vi "PMT_plus_Kiethley2450_and_2410.vi"() -> ()   [LabVIEW 2024]
uses:
  <vilib>/Analysis/NI_AALBase.lvlib
  <vilib>/Analysis/1siggen.llb/Ramp Pattern by Delta.vi
  Keithley 2450/Keithley 2450.lvlib
  archive/Keithley 24XX/Keithley 24XX.lvlib
  <vilib>/Utility/file.llb/Write Delimited Spreadsheet (DBL).vi
  <vilib>/Utility/file.llb/Write Delimited Spreadsheet (string).vi
panel:
  out "Set voltage 2410":dbl
  out "current 2450":dbl format="%e"
  out "actual voltage 2410":dbl format="%0.2f"
  out "current 2410":dbl format="%e"
  in  "Compliance  Level 24210 (0.1)":dbl=0.1
  in  "VISA resource name 2410":refnum<visa-resource-name>
  out "Serial Configuration":T1={"Baud Rate"=9600, "Parity"=0, "Data Bits"=8, "Stop Bits"=10, "Flow Control"=0} {"Flow Control" items=["None", "XON/XOFF", "RTS/CTS", "XON/XOFF & RTS/CTS", "DTR/DSR", "XON/XOFF & DTR/DSR"]; "Stop Bits" items=["1.0"=10, "1.5"=15, "2.0"=20]; "Data Bits" items=["7"=7, "8"=8]; "Parity" items=["None", "Odd", "Even", "Mark", "Space"]; "Baud Rate" items=["300"=300, "600"=600, "1200"=1200, "2400"=2400, "4800"=4800, "9600"=9600, "19200"=19200]}
  in  "Use PMT?":bool=TRUE
  out "XY Graph":cluster{dbl[], dbl[]}(graph)
  out "Actual Voltage 2450":dbl
  in  "Num Current Meas":i32=6
  in  "Path":path
  out "error out":errorcluster
  in  "error in (no error)":errorcluster
  in  "VISA resource name":refnum<visa-resource-name>
  out "Set Voltage 2450":dbl
  in  "Step Size (V)":dbl=0.1 format="%#_13g"
  in  "Max V":dbl format="%#_13g"
  in  "Start V":dbl format="%#_13g"
  in  "Source Limit Level (0.1)":dbl=5e-08
  out "standard deviation":dbl
  out "mean":dbl
  out "data":u32[](array[numeric])
  out "OLD":bool
  out "DB":u32[](array[numeric])
  out "Overload":i32
  out "Gate Number":i32
  in  "Correction":bool=TRUE
  out "Num Gates Read":i32
  out "Gate Time Read":i32 caption="Gate time Read"
  out "Num Gates Set":i32=20
  out "Gate Time Set":i32=200
  out "PowerD":i32 caption="Power\nRead Data"
  out "Handle Number":i32
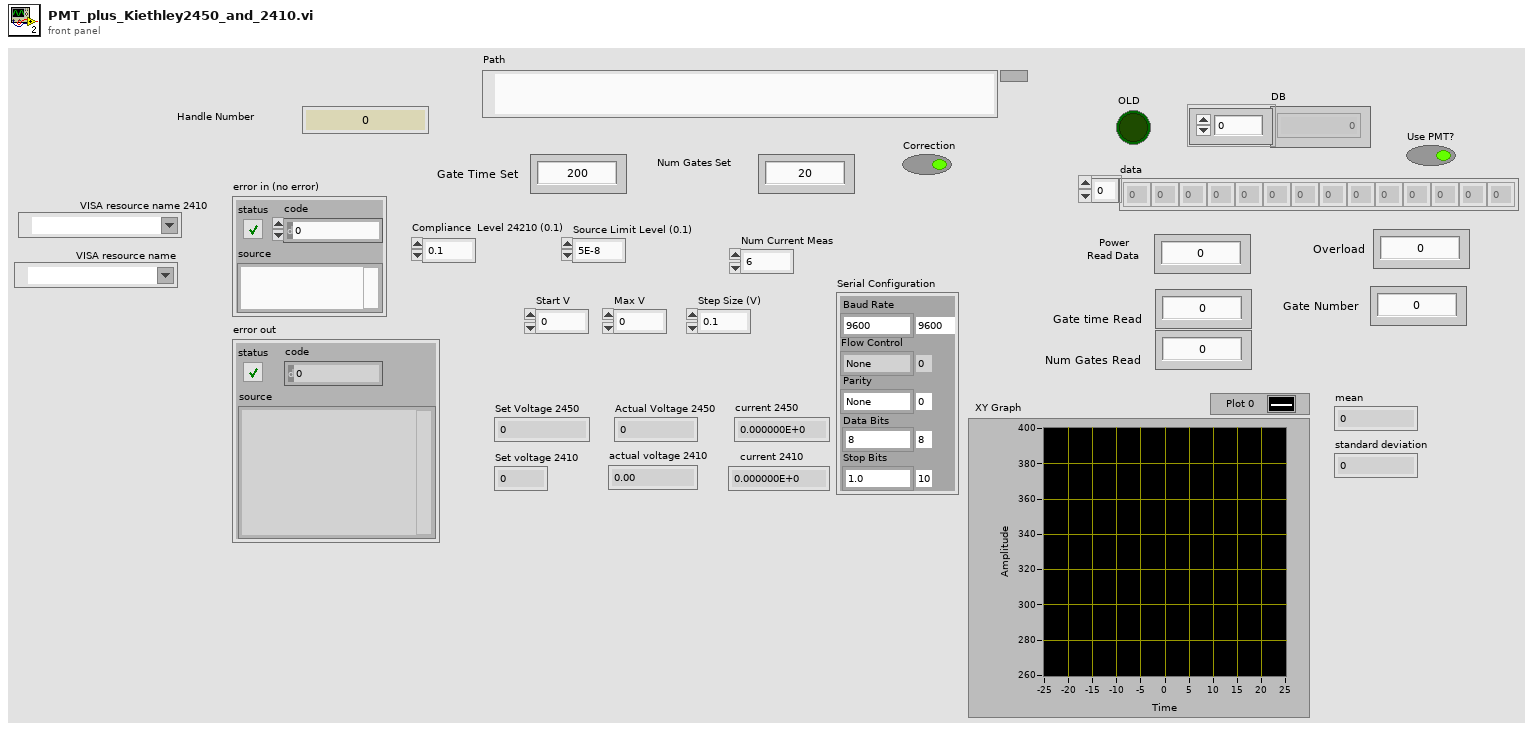
[diagram p1: front panel]
types:
  T1 = cluster{"Baud Rate":u32, "Parity":u16, "Data Bits":u16, "Stop Bits":u16, "Flow Control":u16}
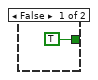
[diagram p2: hidden frame]
diagram:
  n1 = flat-sequence {
    tunnel: [w25] -> w5
    tunnel: [w14] -> w4
    tunnel: [w13] -> w3
    tunnel: ["Path"] -> w1
    tunnel: w5 -> [w43]
    tunnel: w4 -> [w42]
    tunnel: w3 -> [w41]
    tunnel: [w40] -> w2
    tunnel: w1 -> [w39]
    tunnel: w2 -> [w478]
    frame #0 {
      w8 = -1.0
      # "open PMT and turn on power"
      n2 = call "Open.vi"("Serial Number"="30430219") -> ("Handle Number"=w29:i32)  [unwired: 9 in, 1 out]
      "Handle Number" <- w29
      n3 = Boolean To (0,1)(Boolean="Use PMT?") -> (0, 1=w30:i16)
      n4 = call "Read HV.vi"("handle"=w29) -> ("HV out"=w28:i32, "handle out"=w32:i32)  [unwired: 8 in, 1 out]
      n5 = local write "PowerD"(w28) -> ()
      n6 = Multiply(x="Step Size (V)", y=w8) -> (x*y=w6:dbl)
      n7 = Multiply(x="Max V", y=w8) -> (x*y=w16:dbl)
      n8 = To Long Integer(number=w30) -> (32bit integer=w31:i32)
      n9 = call "Set HV.vi"("HV"=w31, "handle"=w32) -> ("handle out"=w34:i32)  [unwired: 8 in, 1 out]
      n10 = call-poly <vilib>:"Ramp Pattern.vi"("start"="Start V", "end"="Max V", "delta"="Step Size (V)") -> ("samples"=w21:i32, "Ramp Pattern"=w18:dbl[])  [unwired: 6 in, 1 out]
      n11 = call-poly <vilib>:"Ramp Pattern.vi"("start"="Max V", "end"=w16, "delta"=w6) -> ("samples"=w22:i32, "Ramp Pattern"=w19:dbl[])  [unwired: 6 in, 1 out]
      n12 = call-poly <vilib>:"Ramp Pattern.vi"("start"=w16, "end"="Start V", "delta"="Step Size (V)") -> ("samples"=w24:i32, "Ramp Pattern"=w20:dbl[])  [unwired: 6 in, 1 out]
      n13 = Add(x=w21, y=w22) -> (x+y=w23:i32)
      n14 = Build Array (concatenate)(w18, w19, w20) -> (w14:dbl[])
      n15 = Build Array("# SetVoltage2450(V) ActualVoltage2450(V) CountsMean CountsStd Current2450(uA) Current2450Std(uA) Current2410(uA) Current2410Std(uA)") -> (w10:string[])
      n16 = call "Read HV.vi"("handle"=w34) -> ("HV out"=w33:i32, "handle out"=w25:i32)  [unwired: 8 in, 1 out]
      n17 = local write "PowerD"(w33) -> ()
      n18 = Add(x=w23, y=w24) -> (x+y=w13:i32)
      n19 = call-poly <vilib>:"Write Delimited Spreadsheet.vi"("file path (dialog if empty)"="Path", "1D data"=w10, "append to file? (new file:F)"=TRUE) -> ()  [unwired: 11 in, 2 out]
    }
    frame #1 {
      w37 = 0
      w38 = 0
      n20 = Initialize Array(w37, w37) -> (w36:i32[])
      n21 = Initialize Array(w38, w38) -> (w35:i32[])
      n22 = for {
        N: w41 -> [_]
        tunnel: w42 -> [w79] mode=indexing
        tunnel: w43 -> [w78]
        tunnel: [w77] -> w40
        tunnel: w39 -> [w76]
        shift-right: [w63] -> _
        shift-left: w35 -> [w71]
        shift-right: [w64] -> _
        shift-left: w36 -> [w70]
        n23 = flat-sequence {
          tunnel: w70 -> [w126]
          tunnel: w71 -> [w127]
          tunnel: w79 -> [w80]
          tunnel: [w80] -> w62
          tunnel: [w127] -> w60
          tunnel: [w126] -> w58
          tunnel: [w110] -> w56
          tunnel: [w109] -> w54
          tunnel: [w93] -> w50
          tunnel: [w92] -> w48
          tunnel: ["Num Current Meas"] -> w46
          tunnel: w62 -> [w135]
          tunnel: [w135] -> w61
          tunnel: w60 -> [w134]
          tunnel: [w134] -> w59
          tunnel: w58 -> [w133]
          tunnel: [w133] -> w57
          tunnel: w56 -> [w132]
          tunnel: [w132] -> w55
          tunnel: w54 -> [w131]
          tunnel: [w131] -> w53
          tunnel: [w130] -> w51
          tunnel: w50 -> [w130]
          tunnel: [w129] -> w49
          tunnel: w48 -> [w129]
          tunnel: [w128] -> w47
          tunnel: w46 -> [w128]
          tunnel: [w169] -> w75
          tunnel: [w170] -> w74
          tunnel: [w140] -> w73
          tunnel: [w169] -> w72
          tunnel: [w168] -> w69
          tunnel: [w167] -> w68
          tunnel: w61 -> [w169]
          tunnel: w59 -> [w168]
          tunnel: w57 -> [w167]
          tunnel: w55 -> [w155]
          tunnel: w53 -> [w156]
          tunnel: [w142] -> w52
          tunnel: w51 -> [w166]
          tunnel: w49 -> [w165]
          tunnel: w47 -> [w152]
          tunnel: [w137] -> w45
          tunnel: [w136] -> w44
          tunnel: w78 -> [w192]
          tunnel: w76 -> [w190]
          tunnel: w75 -> [w189]
          tunnel: w74 -> [w188]
          tunnel: w73 -> [w187]
          tunnel: w72 -> [w185]
          tunnel: w69 -> [w184]
          tunnel: w68 -> [w183]
          tunnel: [w191] -> w67
          tunnel: [w182] -> w66
          tunnel: [w181] -> w65
          tunnel: w52 -> [w180]
          tunnel: w45 -> [w178]
          tunnel: w44 -> [w177]
          tunnel: [w475] -> w63
          tunnel: [w476] -> w64
          tunnel: [w477] -> w77
          tunnel: w67 -> [w477]
          tunnel: w66 -> [w476]
          tunnel: w65 -> [w475]
          frame #0 {
            w95 = u16 0 items=["Voltage", "Current"] ("Source Mode  (0: Voltage)")
            w96 = u16 1 items=["Volts", "Current", "Resistance"] ("Function (0: Volts)")
            w97 = u16 0 items=["Volts", "Current", "Resistance"] ("Function (0: Volts)")
            w102 = TRUE
            w112 = 1
            w114 = 0
            w107 = FALSE
            n24 = Multiply(x=w80, y=-1.0) -> (x*y=w82:dbl)
            "Set voltage 2410" <- w82
            n25 = call "Initialize.vi"("error in (no error)"="error in (no error)", "Reset (True)"=w107, "ID Query (True)"=TRUE, "VISA resource name"="VISA resource name") -> ("error out"=w90:errorcluster, "VISA resource name out"=w91:refnum<visa-resource-name>)  [unwired: 6 in]
            n26 = call "Clear Buffer.vi"("VISA resource name"=w91, "error in (no error)"=w90) -> ("VISA resource name out"=w88:refnum<visa-resource-name>, "error out"=w89:errorcluster)  [unwired: 12 in]
            n27 = call "Configure Measurement Range.vi"("error in (no error)"=w89, "Enable Auto Range (T:Enable)"=w102, "Function (0: Volts)"=w114, "VISA resource name"=w88) -> ("error out"=w124:errorcluster, "VISA resource name out"=w123:refnum<visa-resource-name>)  [unwired: 6 in]
            n28 = call "Initialize.vi"("Reset (True)"=w107, "VISA resource name"="VISA resource name 2410") -> ("error out"=w105:errorcluster, "VISA resource name out"=w106:refnum<visa-resource-name>)  [unwired: 8 in]
            n29 = call "Configure Measurement Range.vi"("error in (no error)"=w124, "Enable Auto Range (T:Enable)"=w102, "Function (0: Volts)"=w112, "VISA resource name"=w123) -> ("error out"=w120:errorcluster, "VISA resource name out"=w117:refnum<visa-resource-name>)  [unwired: 6 in]
            n30 = call "Configure Output.vi"("VISA resource name"=w117, "Source Level (0)"=w80, "Source Limit Level (0.1)"="Source Limit Level (0.1)", "error in (no error)"=w120) -> ("VISA resource name out"=w118:refnum<visa-resource-name>, "error out"=w121:errorcluster)  [unwired: 10 in]
            n31 = call "Configure Measurement.vi"("error in (no error)"=w105, "Enable Auto Range (T:Enable)"=w102, "Function (0: Volts)"=w97, "VISA resource name"=w106) -> ("error out"=w104:errorcluster, "VISA resource name out"=w103:refnum<visa-resource-name>)  [unwired: 6 in]
            n32 = call "Configure Source Function.vi"("error in (no error)"=w121, "Function (0: Volts)"=w114, "VISA resource name"=w118) -> ("error out"=w122:errorcluster, "VISA resource name out"=w119:refnum<visa-resource-name>)  [unwired: 7 in]
            n33 = call "Configure Measurement Function.vi"("error in (no error)"=w122, "Function (0: Volts)"=w112, "VISA resource name"=w119) -> ("error out"=w84:errorcluster, "VISA resource name out"=w87:refnum<visa-resource-name>)  [unwired: 7 in]
            n34 = call "Configure Measurement.vi"("error in (no error)"=w104, "Enable Auto Range (T:Enable)"=w102, "Function (0: Volts)"=w96, "VISA resource name"=w103) -> ("error out"=w100:errorcluster, "VISA resource name out"=w101:refnum<visa-resource-name>)  [unwired: 6 in]
            n35 = call "Set Measurement Count.vi"("error in (no error)"=w84, "Measurement Count"="Num Current Meas", "VISA resource name"=w87) -> ("error out"=w85:errorcluster, "VISA resource name out"=w86:refnum<visa-resource-name>)  [unwired: 7 in]
            n36 = call "Configure Output.vi"("Source Mode  (0: Voltage)"=w95, "error in (no error)"=w100, "Compliance  Level (0.1)"="Compliance  Level 24210 (0.1)", "Output Level (0)"=w82, "VISA resource name"=w101) -> ("error out"=w98:errorcluster, "VISA resource name out"=w99:refnum<visa-resource-name>)  [unwired: 5 in]
            n37 = call "Enable Output.vi"("error in (no error)"=w85, "Enable Output (T: Enable)"=TRUE, "VISA resource name"=w86) -> ("error out"=w110:errorcluster, "VISA resource name out"=w109:refnum<visa-resource-name>)  [unwired: 7 in]
            n38 = call "Enable Output.vi"("error in (no error)"=w98, "VISA resource name"=w99) -> ("error out"=w92:errorcluster, "VISA resource name out"=w93:refnum<visa-resource-name>)  [unwired: 8 in]
            "Set Voltage 2450" <- w80
          }
          frame #1 {
          }
          frame #2 {
            w139 = 1000000
            w164 = u16 0 items=["Fixed", "Sweep", "List"] ("Output Mode (0: Fixed)")
            n39 = call "Make Reading and Store in Buffer.vi"("VISA resource name"=w156, "error in (no error)"=w155) -> ("VISA resource name out"=w154:refnum<visa-resource-name>, "error out"=w153:errorcluster)  [unwired: 12 in]
            n40 = call "Read (Multiple Points).vi"("VISA resource name"=w166, "Sample Count (1)"=w152, "Timeout (10000 ms)"=10000, "error in (no error)"=w165, "Output Mode (0: Fixed)"=w164) -> ("Voltage"=w157:sgl[], "VISA resource name out"=w162:refnum<visa-resource-name>, "Current"=w158:sgl[], "error out"=w159:errorcluster)  [unwired: 4 in, 3 out]
            n41 = call "Read (Multiple Points).vi"("VISA resource name"=w154, "Start Index (1)"=u32 1, "End Index (1)"=w152, "error in (no error)"=w153) -> ("VISA resource name out"=w145:refnum<visa-resource-name>, "Data out"=w150:string, "error out"=w144:errorcluster)  [unwired: 9 in]
            n42 = call <vilib>:"Std Deviation and Variance.vi"("X"=w157) -> ("mean"=→"actual voltage 2410":dbl)  [unwired: 1 in, 2 out]
            n43 = call <vilib>:"Std Deviation and Variance.vi"("X"=w158) -> ("mean"=w137:dbl, "standard deviation"=w136:dbl)  [unwired: 1 in, 1 out]
            "current 2410" <- w137
            n44 = call "Enable Output.vi"("error in (no error)"=w159, "VISA resource name"=w162) -> ("error out"=w160:errorcluster, "VISA resource name out"=w161:refnum<visa-resource-name>)  [unwired: 8 in]
            n45 = call "Close.vi"("error in (no error)"=w160, "VISA resource name"=w161) -> ()  [unwired: 9 in, 1 out]
            n46 = call "Get Source Level.vi"("error in (no error)"=w144, "VISA resource name"=w145) -> ("error out"=w175:errorcluster, "Voltage Level Out"=w170:dbl, "VISA resource name out"=w176:refnum<visa-resource-name>)  [unwired: 6 in, 1 out]
            "Actual Voltage 2450" <- w170
            n47 = Spreadsheet String To Array(delimiter (Tab)=",", format string="%s", spreadsheet string=w150, array type (2D Dbl)=dbl[] []) -> (array=w146:dbl[])
            n48 = call "Enable Output.vi"("error in (no error)"=w175, "Enable Output (T: Enable)"=TRUE, "VISA resource name"=w176) -> ("error out"=w172:errorcluster, "VISA resource name out"=w173:refnum<visa-resource-name>)  [unwired: 7 in]
            n49 = call "Close.vi"("error in (no error)"=w172, "VISA resource name"=w173) -> ("error out"=→"error out":errorcluster)  [unwired: 9 in]
            n50 = call <vilib>:"Std Deviation and Variance.vi"("X"=w146) -> ("mean"=w141:dbl, "standard deviation"=w143:dbl)  [unwired: 1 in, 1 out]
            "current 2450" <- w141
            n51 = Multiply(x=w141, y=w139) -> (x*y=w140:dbl)
            n52 = Multiply(x=w143, y=w139) -> (x*y=w142:dbl)
          }
          frame #3 {
            n53 = case shown="True" FALSE {
              tunnel: [TRUE w196] -> w186
              tunnel: w185 -> [_ w195]
              frame False {
              }
              frame True {
                n54 = Quotient & Remainder(x=w195, y=2) -> (x-y*floor(x/y)=w197:dbl)  [unwired: 1 out]
                n55 = Equal To 0?(x=w197) -> (x = 0?=w196:bool)
              }
            }
            n56 = case shown="True" w186 {
              tunnel: w192 -> [w200 w246]
              tunnel: [w200 w245] -> w191
              tunnel: w190 -> [_ w244]
              tunnel: w189 -> [_ w243]
              tunnel: w188 -> [_ w242]
              tunnel: w187 -> [_ w241]
              tunnel: w184 -> [w199 w240]
              tunnel: w183 -> [w198 w228]
              tunnel: [w199 w216] -> w182
              tunnel: [w198 w215] -> w181
              tunnel: w180 -> [_ w214]
              tunnel: w178 -> [_ w202]
              tunnel: w177 -> [_ w201]
              frame False {
              }
              frame True {
                n57 = flat-sequence {
                  tunnel: [w305] -> w299
                  tunnel: [w303] -> w298
                  tunnel: [w304] -> w297
                  tunnel: w243 -> [w305]
                  tunnel: w242 -> [w304]
                  tunnel: w241 -> [w303]
                  tunnel: w240 -> [w302]
                  tunnel: [w302] -> w229
                  tunnel: w228 -> [w301]
                  tunnel: [w301] -> w221
                  tunnel: w214 -> [w300]
                  tunnel: [w300] -> w210
                  tunnel: [w312] -> w296
                  tunnel: w246 -> [w312]
                  tunnel: [w311] -> w295
                  tunnel: w299 -> [w311]
                  tunnel: [w310] -> w294
                  tunnel: w298 -> [w310]
                  tunnel: [w309] -> w293
                  tunnel: w297 -> [w309]
                  tunnel: [w308] -> w230
                  tunnel: w229 -> [w308]
                  tunnel: [w307] -> w222
                  tunnel: w221 -> [w307]
                  tunnel: [w306] -> w211
                  tunnel: w210 -> [w306]
                  tunnel: w296 -> [w326]
                  tunnel: [w321] -> w292
                  tunnel: [w319] -> w291
                  tunnel: w295 -> [w319]
                  tunnel: [w318] -> w290
                  tunnel: w294 -> [w318]
                  tunnel: [w317] -> w289
                  tunnel: w293 -> [w317]
                  tunnel: [w316] -> w231
                  tunnel: w230 -> [w316]
                  tunnel: [w315] -> w223
                  tunnel: w222 -> [w315]
                  tunnel: [w314] -> w212
                  tunnel: w211 -> [w314]
                  tunnel: [w335] -> w288
                  tunnel: w292 -> [w337]
                  tunnel: [w332] -> w287
                  tunnel: w291 -> [w332]
                  tunnel: w290 -> [w331]
                  tunnel: [w331] -> w286
                  tunnel: [w330] -> w285
                  tunnel: w289 -> [w330]
                  tunnel: [w329] -> w232
                  tunnel: w231 -> [w329]
                  tunnel: [w328] -> w224
                  tunnel: w223 -> [w328]
                  tunnel: [w327] -> w213
                  tunnel: w212 -> [w327]
                  tunnel: w288 -> [w350]
                  tunnel: [w350] -> w284
                  tunnel: [w346] -> w283
                  tunnel: [w346] -> w282
                  tunnel: [w345] -> w281
                  tunnel: w287 -> [w345]
                  tunnel: [w344] -> w280
                  tunnel: w286 -> [w344]
                  tunnel: w285 -> [w343]
                  tunnel: [w343] -> w279
                  tunnel: [w342] -> w233
                  tunnel: w232 -> [w342]
                  tunnel: [w341] -> w225
                  tunnel: w224 -> [w341]
                  tunnel: w213 -> [w340]
                  tunnel: [w340] -> w206
                  tunnel: w284 -> [w363]
                  tunnel: [w359] -> w278
                  tunnel: w283 -> [w358]
                  tunnel: w282 -> [w357]
                  tunnel: [w358] -> w277
                  tunnel: [w357] -> w276
                  tunnel: w281 -> [w356]
                  tunnel: [w356] -> w275
                  tunnel: [w355] -> w274
                  tunnel: w280 -> [w355]
                  tunnel: [w354] -> w273
                  tunnel: w279 -> [w354]
                  tunnel: [w353] -> w234
                  tunnel: w233 -> [w353]
                  tunnel: [w352] -> w226
                  tunnel: w225 -> [w352]
                  tunnel: [w351] -> w207
                  tunnel: w206 -> [w351]
                  tunnel: [w376] -> w272
                  tunnel: w278 -> [w375]
                  tunnel: w277 -> [w374]
                  tunnel: w276 -> [w373]
                  tunnel: [w372] -> w271
                  tunnel: [w369] -> w270
                  tunnel: w275 -> [w369]
                  tunnel: [w368] -> w269
                  tunnel: w274 -> [w368]
                  tunnel: w273 -> [w367]
                  tunnel: [w367] -> w268
                  tunnel: [w366] -> w235
                  tunnel: w234 -> [w366]
                  tunnel: [w365] -> w227
                  tunnel: w226 -> [w365]
                  tunnel: [w364] -> w208
                  tunnel: w207 -> [w364]
                  tunnel: w272 -> [w430]
                  tunnel: [w429] -> w267
                  tunnel: [w428] -> w266
                  tunnel: w271 -> [w428]
                  tunnel: w270 -> [w427]
                  tunnel: [w427] -> w265
                  tunnel: [w426] -> w264
                  tunnel: w269 -> [w426]
                  tunnel: [w425] -> w263
                  tunnel: w268 -> [w425]
                  tunnel: [w424] -> w236
                  tunnel: w235 -> [w424]
                  tunnel: w227 -> [w423]
                  tunnel: [w423] -> w218
                  tunnel: [w422] -> w209
                  tunnel: w208 -> [w422]
                  tunnel: w267 -> [w437]
                  tunnel: w266 -> [w438]
                  tunnel: [w438] -> w262
                  tunnel: [w437] -> w261
                  tunnel: [w436] -> w260
                  tunnel: w265 -> [w436]
                  tunnel: w264 -> [w435]
                  tunnel: [w435] -> w259
                  tunnel: w263 -> [w434]
                  tunnel: [w434] -> w258
                  tunnel: [w433] -> w237
                  tunnel: w236 -> [w433]
                  tunnel: [w432] -> w219
                  tunnel: w218 -> [w432]
                  tunnel: w209 -> [w431]
                  tunnel: [w431] -> w203
                  tunnel: [w446] -> w257
                  tunnel: w262 -> [w446]
                  tunnel: [w445] -> w256
                  tunnel: w261 -> [w445]
                  tunnel: [w444] -> w255
                  tunnel: w260 -> [w444]
                  tunnel: [w443] -> w254
                  tunnel: w259 -> [w443]
                  tunnel: [w442] -> w253
                  tunnel: w258 -> [w442]
                  tunnel: [w441] -> w238
                  tunnel: w237 -> [w441]
                  tunnel: [w440] -> w220
                  tunnel: w219 -> [w440]
                  tunnel: [w439] -> w204
                  tunnel: w203 -> [w439]
                  tunnel: w257 -> [w456]
                  tunnel: [w455] -> w252
                  tunnel: [w454] -> w251
                  tunnel: [w453] -> w250
                  tunnel: w256 -> [w453]
                  tunnel: [w452] -> w249
                  tunnel: w255 -> [w452]
                  tunnel: [w451] -> w248
                  tunnel: w254 -> [w451]
                  tunnel: [w450] -> w247
                  tunnel: w253 -> [w450]
                  tunnel: [w449] -> w239
                  tunnel: w238 -> [w449]
                  tunnel: w220 -> [w448]
                  tunnel: [w448] -> w217
                  tunnel: [w447] -> w205
                  tunnel: w204 -> [w447]
                  tunnel: w252 -> [w463]
                  tunnel: w251 -> [w471]
                  tunnel: [w473] -> w245
                  tunnel: w250 -> [w473]
                  tunnel: w244 -> [w472]
                  tunnel: w249 -> [w466]
                  tunnel: w248 -> [w469]
                  tunnel: w247 -> [w462]
                  tunnel: w239 -> [w465]
                  tunnel: w217 -> [w464]
                  tunnel: [w461] -> w216
                  tunnel: [w460] -> w215
                  tunnel: w205 -> [w459]
                  tunnel: w202 -> [w458]
                  tunnel: w201 -> [w457]
                  frame #0 {
                  }
                  frame #1 {
                    n58 = Wait (ms)(milliseconds to wait=u32 200) -> ()  [unwired: 1 out]
                  }
                  frame #2 {
                    # "set gate time"
                    n59 = local read "Gate Time Set"() -> (w323:i32)
                    n60 = Wait (ms)(milliseconds to wait=u32 200) -> ()  [unwired: 1 out]
                    n61 = To Long Integer(number=w323) -> (32bit integer=w324:i32)
                    n62 = call "Set IT.vi"("IT"=w324, "handle"=w326) -> ("handle out"=w325:i32)  [unwired: 8 in, 1 out]
                    n63 = call "Read IT.vi"("handle"=w325) -> ("IT out"=w322:i32, "handle out"=w321:i32)  [unwired: 8 in, 1 out]
                    n64 = local write "Gate Time Read"(w322) -> ()
                  }
                  frame #3 {
                    # "set number of gates"
                    n65 = local read "Num Gates Set"() -> (w339:i32)
                    n66 = Wait (ms)(milliseconds to wait=u32 200) -> ()  [unwired: 1 out]
                    n67 = To Long Integer(number=w339) -> (32bit integer=w338:i32)
                    n68 = call "Set RN.vi"("RN"=w338, "handle"=w337) -> ("handle out"=w336:i32)  [unwired: 8 in, 1 out]
                    n69 = call "Read RN.vi"("handle"=w336) -> ("RN out"=w334:i32, "handle out"=w335:i32)  [unwired: 8 in, 1 out]
                    n70 = local write "Num Gates Read"(w334) -> ()
                  }
                  frame #4 {
                    # "gate number data"
                    # "count data"
                    n71 = local write "Gate Number"(0) -> ()
                    n72 = Initialize Array(u32 0, 0 ("次元サイズ")) -> (w346:u32[])
                  }
                  frame #5 {
                    n73 = Boolean To (0,1)(Boolean="Correction") -> (0, 1=w362:i16)
                    n74 = To Long Integer(number=w362) -> (32bit integer=w361:i32)
                    n75 = call "Count Start.vi"("Correction"=w361, "handle"=w363) -> ("handle out"=w359:i32)  [unwired: 8 in, 1 out]
                  }
                  frame #6 {
                    n76 = local read "Num Gates Read"() -> (w371:i32)
                    n77 = for {
                      N: w371 -> [_]
                      shift-right: [w377] -> w372
                      shift-left: w374 -> [w385]
                      shift-right: [w381] -> _
                      shift-left: w373 -> [w384]
                      tunnel: w375 -> [w386]
                      tunnel: [w387] -> w376
                      tunnel: [w377] -> w370
                      n78 = flat-sequence {
                        tunnel: [w397] -> w391
                        tunnel: [w396] -> w382
                        tunnel: [w395] -> w379
                        tunnel: w386 -> [w397]
                        tunnel: w385 -> [w396]
                        tunnel: w384 -> [w395]
                        tunnel: [w408] -> w390
                        tunnel: w391 -> [w407]
                        tunnel: [w402] -> w389
                        tunnel: [w401] -> w388
                        tunnel: [w400] -> w383
                        tunnel: w382 -> [w400]
                        tunnel: [w399] -> w380
                        tunnel: w379 -> [w399]
                        tunnel: [w398] -> w378
                        tunnel: w390 -> [w421]
                        tunnel: w389 -> [w416]
                        tunnel: w388 -> [w415]
                        tunnel: w383 -> [w413]
                        tunnel: w380 -> [w412]
                        tunnel: w378 -> [w411]
                        tunnel: [w421] -> w387
                        tunnel: [w414] -> w377
                        tunnel: [w409] -> w381
                        frame #0 {
                          n79 = Initialize Array(u32 0, 16 ("次元サイズ")) -> (w392:u32[])
                          n80 = local write "DB"(w392) -> ()
                        }
                        frame #1 {
                          # "read data"
                          n81 = local read "Gate Number"() -> (w406:i32)
                          n82 = local read "Overload"() -> (w405:i32)
                          n83 = local read "DB"() -> (w403:u32[])
                          n84 = call "Read Data.vi"("OLD"=w405, "DataBuf"=w403, "GateNum"=w406, "handle"=w407) -> ("OLD out"=w404:i32, "DataBuf out"=w401:u32[], "GateNum out"=w398:i32, "handle out"=w408:i32, "function return"=w402:u32)  [unwired: 3 in]
                          n85 = local write "Gate Number"(w398) -> ()
                          n86 = local write "DB"(w401) -> ()
                          n87 = local write "Overload"(w404) -> ()
                        }
                        frame #2 {
                          # "Pickup Tans Data!"
                          n88 = To Long Integer(number=w416) -> (32bit integer=w417:i32)
                          n89 = Build Array(w411) -> (w410:i32[])
                          n90 = local read "Overload"() -> (w419:i32)
                          n91 = Build Array (concatenate)(w412, w410) -> (w409:u32[])
                          n92 = Not Equal To 0?(x=w419) -> (x != 0?=→"OLD":bool)
                          n93 = Array Subset(array=w415, length=w417) -> (w418:u32[])  [unwired: 1 in]
                          n94 = Build Array (concatenate)(w413, w418) -> (w414:u32[])
                        }
                      }
                    }
                    "data" <- w370
                  }
                  frame #7 {
                    # "data"
                    n95 = call "Count Stop.vi"("handle"=w430) -> ("handle out"=w429:i32)  [unwired: 9 in, 1 out]
                  }
                  frame #8 {
                  }
                  frame #9 {
                  }
                  frame #10 {
                    n96 = call <vilib>:"Std Deviation and Variance.vi"("X"=w456) -> ("mean"=w455:dbl, "standard deviation"=w454:dbl)  [unwired: 1 in, 1 out]
                  }
                  frame #11 {
                    n97 = Build Array (concatenate)(w464, w462) -> (w461:dbl[])
                    n98 = Build Array (concatenate)(w465, w463) -> (w460:dbl[])
                    n99 = Build Array(w466, w462, w463, w471, w469, w459, w458, w457) -> (w470:dbl[])
                    n100 = call-poly <vilib>:"Write Delimited Spreadsheet.vi"("file path (dialog if empty)"=w472, "format (%.3f)"="%.10f", "1D data"=w470, "append to file? (new file:F)"=TRUE) -> ()  [unwired: 10 in, 2 out]
                    "mean" <- w463
                    "standard deviation" <- w471
                  }
                }
              }
            }
          }
          frame #4 {
            n101 = Bundle(w476, w475) -> (→"XY Graph":cluster{dbl[], dbl[]})  [unwired: 1 in]
          }
        }
      }
    }
    frame #2 {
      # "turn off PMT and close"
      n102 = Boolean To (0,1)(Boolean=FALSE) -> (0, 1=w483:i16)
      n103 = To Long Integer(number=w483) -> (32bit integer=w482:i32)
      n104 = call "Set HV.vi"("HV"=w482, "handle"=w478) -> ("handle out"=w480:i32)  [unwired: 8 in, 1 out]
      n105 = call "Read HV.vi"("handle"=w480) -> ("HV out"=w484:i32, "handle out"=w479:i32)  [unwired: 8 in, 1 out]
      n106 = call "Close.vi"("Handle"=w479) -> ()  [unwired: 9 in, 2 out]
      n107 = local write "PowerD"(w484) -> ()
    }
  }
